vi "picoharp_write_header.vi"(8 "error in (no error)":errorcluster, 11 "hydraharp in":refnum<class "picoharp.lvclass">) -> (0 "error out":errorcluster, 3 "hydraharp out":refnum<class "picoharp.lvclass">)   [LabVIEW 2015, in "picoharp.lvclass"]
uses:
  picoharp.lvclass
  picoharp.lvclass/picoharp.ctl
  Hydraharp/hdf5_photon_record_logger/stream_metadata.ctl
  Hydraharp/hydraharp_panel/hpanel_hydraharp_settings.ctl
  Hydraharp/hydraharp_panel/hpanel_sync_settings.ctl
  Hydraharp/hydraharp_panel/hpanel_sync_div.ctl
  Hydraharp/hydraharp_panel/hpanel_channel_settings.ctl
  Data Logger Class/data_logger.lvclass
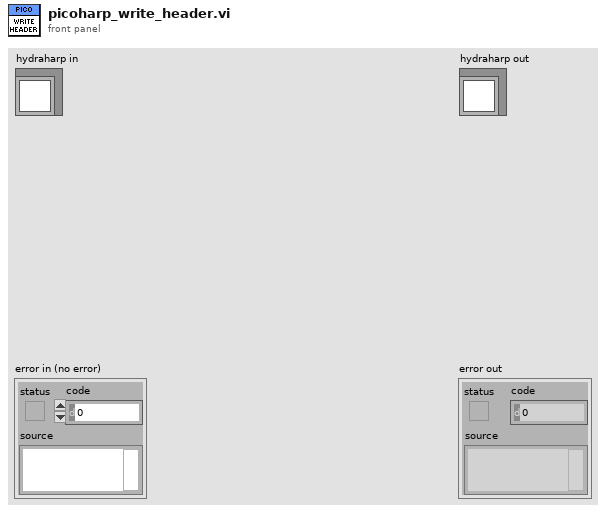
[diagram p1: front panel]
types:
  T1 = typedef "stream_metadata.ctl" = cluster{"Hydraharp Settings":T2, "resolution":dbl, "stream_notes":string}
  T2 = typedef "hpanel_hydraharp_settings.ctl" = cluster{"Sync Settings":T3, "CH 1":T5, "CH 2":T5, "CH 3":T5, "CH 4":T5, "binning":i32, "CH 5":T5, "CH 6":T5, "CH 7":T5, "CH 8":T5}
  T3 = typedef "hpanel_sync_settings.ctl" = cluster{"snc_count":i32, "snc_level":i32, "snc_ZeroX":i32, "snc_offs":i32, "sync_div":T4}
  T4 = typedef "hpanel_sync_div.ctl" = enum16{"1", "2", "4", "8"}
  T5 = typedef "hpanel_channel_settings.ctl" = cluster{"ch_counts":i32, "ch_level":i32, "ch_ZeroX":i32, "ch_offs":i32}
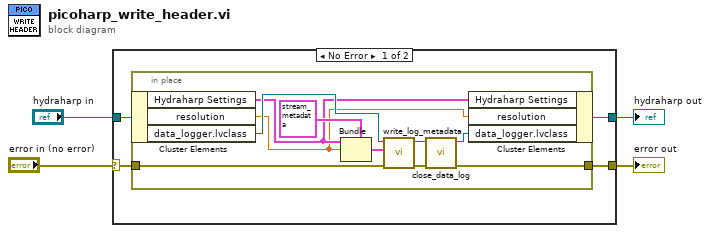
[diagram p0: block diagram]
diagram:
  n1 = case shown="No Error" "error in (no error)" {
    selector: "error in (no error)" -> [w8 w20]
    tunnel: [w5 w20] -> w3
    tunnel: [w6 w19] -> w1
    tunnel: "hydraharp in" -> [w7 w19]
    frame No Error {
      n2 = in-place {
        in-place-border: w8 -> [w13]
        in-place-border: [w9] -> w5
        n3 = in-place-cluster #1(w7) -> ("Hydraharp Settings"=w16:T2, "resolution"=w15:dbl, "data_logger.lvclass"=w18:refnum<class "data_logger.lvclass">)
        n4 = Bundle(cluster=T1 {"Hydraharp Settings"={"Sync Settings"={"snc_count"=0, "snc_level"=0, "snc_ZeroX"=0, "snc_offs"=0, "sync_div"=enum."1"}, "CH 1"={"ch_counts"=0, "ch_level"=0, "ch_ZeroX"=0, "ch_offs"=0}, "CH 2"={"ch_counts"=0, "ch_level"=0, "ch_ZeroX"=0, "ch_offs"=0}, "CH 3"={"ch_counts"=0, "ch_level"=0, "ch_ZeroX"=0, "ch_offs"=0}, "CH 4"={"ch_counts"=0, "ch_level"=0, "ch_ZeroX"=0, "ch_offs"=0}, "binning"=0, "CH 5"={"ch_counts"=0, "ch_level"=0, "ch_ZeroX"=0, "ch_offs"=0}, "CH 6"={"ch_counts"=0, "ch_level"=0, "ch_ZeroX"=0, "ch_offs"=0}, "CH 7"={"ch_counts"=0, "ch_level"=0, "ch_ZeroX"=0, "ch_offs"=0}, "CH 8"={"ch_counts"=0, "ch_level"=0, "ch_ZeroX"=0, "ch_offs"=0}}, "resolution"=0.0, "stream_notes"="stream_notes"} ("output cluster"), "Hydraharp Settings"=w16, "resolution"=w15) -> (w14:T1)  [unwired: 1 in]
        n5 = call-dynamic "write_log_metadata.vi"("error in (no error)"=w13, "data"=w14, "data_logger in"=w18) -> ("error out"=w10:errorcluster, "data_logger out"=w12:refnum<class "data_logger.lvclass">)  [unwired: 7 in]
        n6 = call-dynamic "close_data_log.vi"("error in (no error)"=w10, "data_logger in"=w12) -> ("error out"=w9:errorcluster, "data_logger out"=w11:refnum<class "data_logger.lvclass">)  [unwired: 8 in]
        n7 = in-place-cluster #1("Hydraharp Settings"=w16, "resolution"=w15, "data_logger.lvclass"=w11) -> (w6:refnum<class "picoharp.lvclass">)
      }
    }
    frame Error {
    }
  }
  "error out" <- w3
  "hydraharp out" <- w1
